vi "KE2000_Test.vi"(8 "error in (no error)":errorcluster, 11 "KE2000 in":refnum<class "KE2000.lvclass">) -> (0 "error out":errorcluster, 3 "KE2000 out":refnum<class "KE2000.lvclass">)   [LabVIEW 2013, in "KE2000.lvclass"]
uses:
  KE2000.lvclass
  <vilib>/Platform/TimedLoop/XDataNode/timing_clust.ctl
  <vilib>/Platform/TimedLoop/XDataNode/nitl_modes.ctl
  <vilib>/Platform/TimedLoop/XDataNode/wakeup.ctl
  InstrumentSetup.vi
  <vilib>/platform/TimedLoop/XDataNode/XDataNode.xnode
  InstrControl.lvclass
  <vilib>/Platform/TimedLoop/XDataNode/XDNodeRunTimeDep.lvlib
panel:
  out "Numeric":dbl
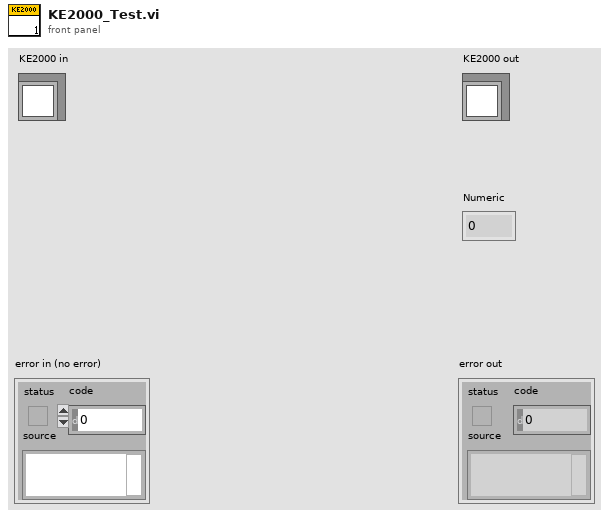
[diagram p1: front panel]
types:
  T1 = cluster{"KE 2410":cluster{"Instrument name":string, "address":refnum<visa-resource-name>, "Instrument type":u16}, "KE 2410_2":cluster{"Instrument name":string, "address":refnum<visa-resource-name>, "Instrument type":u16}, "KE 6517":cluster{"Instrument name":string, "address":refnum<visa-resource-name>, "Instrument type":u16}, "KE 6517_2":cluster{"Instrument name":string, "address":refnum<visa-resource-name>, "Instrument type":u16}, "KE 487":cluster{"Instrument name":string, "address":refnum<visa-resource-name>, "Instrument type":u16}, "KE 236":cluster{"Instrument name":string, "address":refnum<visa-resource-name>, "Instrument type":u16}, "WK 6440B":cluster{"Instrument name":string, "address":refnum<visa-resource-name>, "Instrument type":u16}, "WK 6425":cluster{"Instrument name":string, "address":refnum<visa-resource-name>, "Instrument type":u16}, "HP 4263B":cluster{"Instrument name":string, "address":refnum<visa-resource-name>, "Instrument type":u16}, "Pickering Matrix":cluster{"Instrument name":string, "address":refnum<visa-resource-name>, "Instrument type":u16}, "KE 2000":cluster{"Instrument name":string, "address":refnum<visa-resource-name>, "Instrument type":u16}, "KE3706A Switching":cluster{"Instrument name":string, "address":refnum<visa-resource-name>, "Instrument type":u16}}
  T2 = cluster{"Range":u16, "Range Value":dbl, "Function":u16, "KE2000":refnum<class "KE2000.lvclass">}
  T3 = typedef "XDNodeRunTimeDep.lvlib/timing_clust.ctl" = cluster{"Expected End [f-1]":u64, "Actual End [f-1]":u64, "Finished Late? [f-1]":bool, "Expected End [i-1]":u64, "Actual End [i-1]":u64, "Finished Late? [i-1]":bool, "Expected Start [i]":u64, "Actual Start [i]":u64, "Expected Start [f]":u64, "Actual Start [f]":u64, "Source Name":string, "Structure Name":string, "Period":i64, "Deadline":i64, "Offset":i64, "Start":i64, "Priority":i32, "Timeout":i32, "Mode":T4, "Wakeup Reason":T5, "Error":errorcluster, "Source Type":string, "Secondary Source Type":string, "Global End Time":u64, "Global Start Time":u64, "Frame Duration":u64, "Iteration Duration":u64, "Assigned CPU":i32, "I/O Scan Engine Mode":u32}
  T4 = typedef "XDNodeRunTimeDep.lvlib/nitl_modes.ctl" = enum32{"No Change", "Process missed periods, maintain original phase", "Discard missed periods, maintain original phase", "Process missed periods, ignore original phase", "Discard missed periods, ignore original phase"}
  T5 = typedef "XDNodeRunTimeDep.lvlib/wakeup.ctl" = enum32{"Normal", "Aborted", "Asynchronous wakeup", "Timing source error", "Timed loop error", "Timeout"}
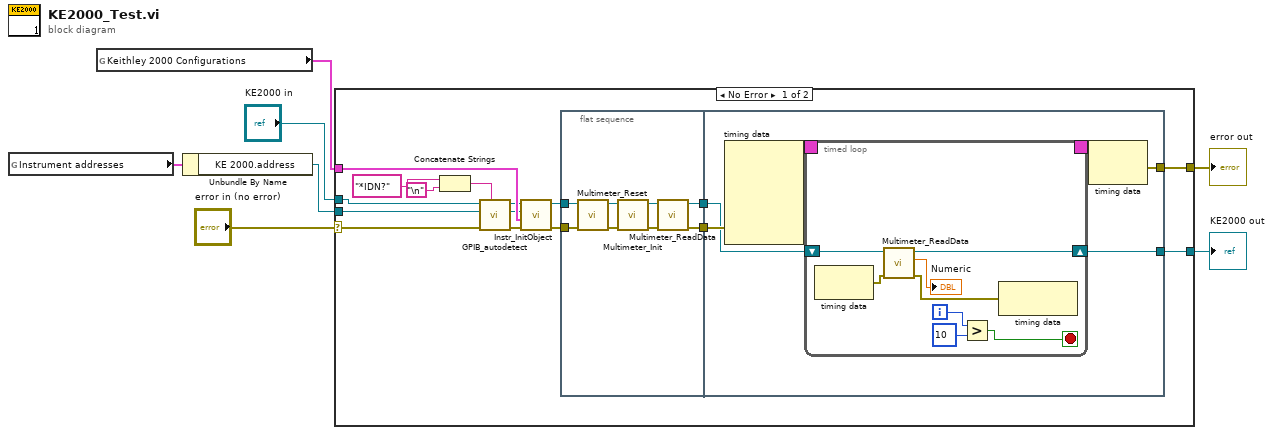
[diagram p0: block diagram]
diagram:
  n1 = global read "InstrumentSetup.vi" "Instrument addresses"() -> (w3:T1)
  n2 = global read "InstrumentSetup.vi" "Keithley 2000 Configurations"() -> (w2:T2)
  n3 = Unbundle By Name(w3) -> ("KE 2000.address"=w1:refnum<visa-resource-name>)
  n4 = case shown="No Error" "error in (no error)" {
    selector: "error in (no error)" -> [w19 w57]
    tunnel: [w10 w57] -> w6
    tunnel: [w11 w56] -> w4
    tunnel: "KE2000 in" -> [w20 w56]
    tunnel: w2 -> [w17 _]
    tunnel: w1 -> [w18 _]
    frame No Error {
      n5 = Concatenate Strings("*IDN?" ("regular expression"), "\n") -> (w21:string)
      n6 = call-dynamic "GPIB_autodetect.vi"("ID command"=w21, "error in (no error)"=w19, "Instrument address in"=w18, "InstrControl in"=w20) -> ("error out"=w14:errorcluster, "Instrument address out"=w16:refnum<visa-resource-name>, "InstrControl out"=w15:refnum<class "KE2000.lvclass">)  [unwired: 5 in]
      n7 = call-dynamic "Instr_InitObject.vi"("error in (no error)"=w14, "Instrument Configuration"=w17, "Instrument address"=w16, "KE2000 in"=w15) -> ("error out"=w13:errorcluster, "KE2000 out"=w12:refnum<class "KE2000.lvclass">)  [unwired: 6 in]
      n8 = flat-sequence {
        tunnel: w13 -> [w27]
        tunnel: w12 -> [w26]
        tunnel: [w25] -> w9
        tunnel: [w24] -> w8
        tunnel: [w35] -> w11
        tunnel: [w34] -> w10
        tunnel: w9 -> [w33]
        tunnel: w8 -> [w32]
        frame #0 {
          n9 = call-dynamic "Multimeter_Reset.vi"("error in (no error)"=w27, "MultimeterControl in"=w26) -> ("error out"=w30:errorcluster, "MultimeterControl out"=w31:refnum<class "KE2000.lvclass">)  [unwired: 8 in]
          n10 = call-dynamic "Multimeter_Init.vi"("error in (no error)"=w30, "MultimeterControl in"=w31) -> ("error out"=w28:errorcluster, "MultimeterControl out"=w29:refnum<class "KE2000.lvclass">)  [unwired: 8 in]
          n11 = call-dynamic "Multimeter_ReadData.vi"("error in (no error)"=w28, "MultimeterControl in"=w29) -> ("error out"=w25:errorcluster, "MultimeterControl out"=w24:refnum<class "KE2000.lvclass">)  [unwired: 7 in, 1 out]
        }
        frame #1 {
          n12 = node-c288(w33) -> (w37:T3)  [unwired: 4 in]
          n13 = timed-loop {
            timing: w37 -> [_]
            timing-out: [_] -> w36
            shift-right: [w41] -> w35
            shift-left: w32 -> [w40]
            i -> [w44]
            stop <- w43 stop-if-true
            n14 = node-c288() -> (w39:errorcluster)  [unwired: 1 in]
            n15 = call-dynamic "Multimeter_ReadData.vi"("error in (no error)"=w39, "MultimeterControl in"=w40) -> ("error out"=w38:errorcluster, "Voltage in V"=→"Numeric":dbl, "MultimeterControl out"=w41:refnum<class "KE2000.lvclass">)  [unwired: 7 in]
            n16 = Greater?(x=w44, y=10) -> (0:w43:bool)
            n17 = node-c288(w38) -> ()  [unwired: 1 out]
          }
          n18 = node-c288(w36) -> (w34:errorcluster)
        }
      }
    }
    frame Error {
    }
  }
  "error out" <- w6
  "KE2000 out" <- w4
